vi "寄存器值更新.vi"(0 "MainPage输入":refnum<class "MainPage.lvclass">, 1 "NewVal":u16[](array[numeric])) -> ()   [LabVIEW 2019, in "MainPage.lvlib" / "MainPage.lvclass"]
uses:
  MainPage.lvclass
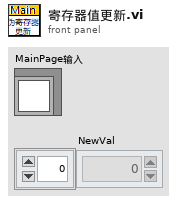
[diagram p1: front panel]
types:
  T1 = typedef "MainPage.lvlib/MainPage.lvclass/DataRef_通讯接口.ctl" = cluster{"连接方式":enum16{"网口(客服端)", "网口(服务端)", "串口"}, "VISA串口名称":refnum<visa-resource-name>, "服务端识别":cluster{"本机IP":string, "本机端口":u16, "当前目标":string}, "客服端识别":cluster{"客P-主IP:Port":string}, "服务端记录":cluster{"服务端侦听ID":refnum<k5>, "服务端接口记录":map{string, refnum<k5>}}, "客服端记录":map{string, refnum<k5>}}
  T2 = cluster{"寄存器模拟":u16[], "串口正常？":bool, "报文信息记录":string[][]}
  T3 = enum16{"ini", "增加记录", "读取记录", "更改寄存器值", "更改接口状态", "更改报文信息", "增加报文信息"}
  T4 = cluster{"串口正常？":bool, "寄存器模拟":u16[], "报文信息记录":string[][]}
  T5 = enum16{"ini", "读取", "写入-报文记录", "写入-寄存器模拟", "写入-串口状态", "增加报文记录"}
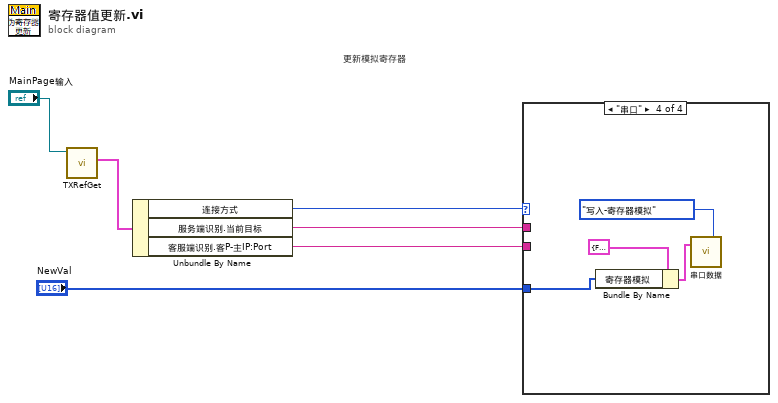
[diagram p0: block diagram]
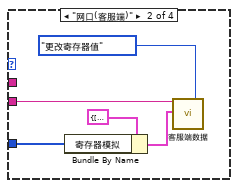
[diagram p3: hidden frame]
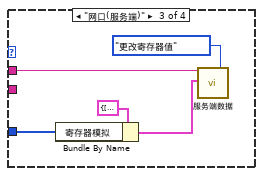
[diagram p4: hidden frame]
diagram:
  # "更新模拟寄存器"
  n1 = call-dynamic "TXRefGet.vi"("MainPage 输入"="MainPage输入") -> ("通讯接口数据"=w2:T1)  [unwired: 6 in, 4 out]
  n2 = Unbundle By Name(w2) -> ("连接方式"=w3:enum16{"网口(客服端)", "网口(服务端)", "串口"}, "服务端识别.当前目标"=w5:string, "客服端识别.客P-主IP:Port"=w4:string)
  n3 = case shown="\"串口\"" w3 {
    tunnel: w4 -> [_ w9 _ _]
    tunnel: w5 -> [_ _ w14 _]
    tunnel: "NewVal" -> [_ w11 w16 w18]
    frame Default {
    }
    frame "网口(客服端)" {
      n4 = Bundle By Name(cluster=T2 {"寄存器模拟"=[], "串口正常？"=FALSE, "报文信息记录"=[]} ("数据输入"), "寄存器模拟"=w11) -> (w7:T2)
      n5 = call "客服端数据.vi"("客P-主IP:P"=w9, "数据输入"=w7, "枚举"=T3."更改寄存器值") -> ()  [unwired: 15 in, 2 out]
    }
    frame "网口(服务端)" {
      n6 = Bundle By Name(cluster=T2 {"寄存器模拟"=[], "串口正常？"=FALSE, "报文信息记录"=[]} ("数据输入"), "寄存器模拟"=w16) -> (w12:T2)
      n7 = call "服务端数据.vi"("IP-Port"=w14, "数据输入"=w12, "枚举"=T3."更改寄存器值") -> ()  [unwired: 15 in, 2 out]
    }
    frame "串口" {
      n8 = Bundle By Name(cluster=T4 {"串口正常？"=FALSE, "寄存器模拟"=[], "报文信息记录"=[]} ("串口输入"), "寄存器模拟"=w18) -> (w17:T4)
      n9 = call "串口数据.vi"("串口输入"=w17, "枚举"=T5."写入-寄存器模拟") -> ()  [unwired: 17 in, 1 out]
    }
  }
